vi "Distance Sensor.vi"(8 "error in (no error)":errorcluster) -> (0 "error out":errorcluster, 2 "Distance 2":dbl)   [LabVIEW 2016]
uses:
  <vilib>/Rock Robotics/WPI/Ultrasonic/WPI_SonarMB1010AnalogRefNum Registry Get.vi
  <vilib>/Rock Robotics/WPI/Ultrasonic/WPI_SonarMB1010AnalogGetRange.vi
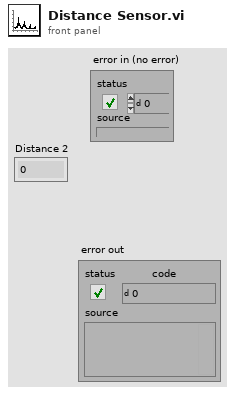
[diagram p1: front panel]
types:
  T1 = typedef "WPI_SonarMB1010AnalogDeviceRef.ctl" = cluster{"AIDeviceRef":T2, "Scaling factor (V/in)":dbl, "Average Bits":u8}
  T2 = typedef "WPI_AnalogChannelDevRef.ctl" = cluster{"DevStatus":errorcluster, "Analog Channel":T3}
  T3 = typedef "FPGA_AIChannel.ctl" = enum8{"AI 0", "AI 1", "AI 2", "AI 3", "AI MXP 0", "AI MXP 1", "AI MXP 2", "AI MXP 3", "Invalid"}
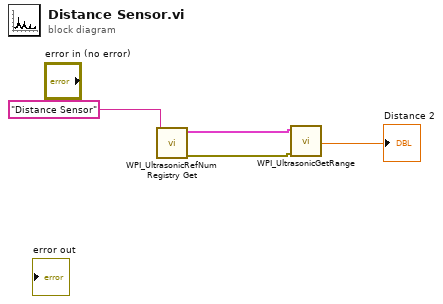
[diagram p0: block diagram]
diagram:
  n1 = call-poly <vilib>:"WPI_UltrasonicRefNum Registry Get.vi"("refnum name"="Distance Sensor") -> ("error out"=w1:errorcluster, "SonarMB1010AnalogDevRef"=w3:T1)  [unwired: 9 in]
  n2 = call-poly <vilib>:"WPI_UltrasonicGetRange.vi"("error in"=w1, "SonarMB1010AnalogDevRef"=w3) -> ("Distance"=→"Distance 2":dbl)  [unwired: 7 in, 2 out]
